vi "DAC set.vi"(1 "DAC number":u8=1 min=1 max=8, 2 "DAC set [mV]":dbl=-720.0, 3 "DAC COM port":refnum<visa-resource-name>="COM3") -> (0 "DAC read (mV)":dbl)   [LabVIEW 2011]
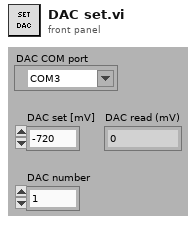
[diagram p1: front panel]
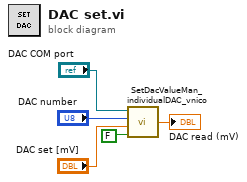
[diagram p0: block diagram]
diagram:
  n1 = call "SetDacValueMan_individualDAC_vnico.vi"("DAC"=FALSE, "DAC write (mV)"="DAC set [mV]", "DAC number"="DAC number", "RS232/ Optical Fiber"="DAC COM port") -> ("DAC read (mV)"=→"DAC read (mV)":dbl)
